vi "FTW-Collection-KeyValue-JSON-Serialize.vi"(1 "Key-Value Pair":T1) -> (0 "Serialized Key-Value Pair":string)   [LabVIEW 2014]
uses:
  FTW-Collection-KeyValuePair.ctl
  JSON/FTW-JSON-Escape.vi
panel:
  # "Inputs"
  # "Outputs"
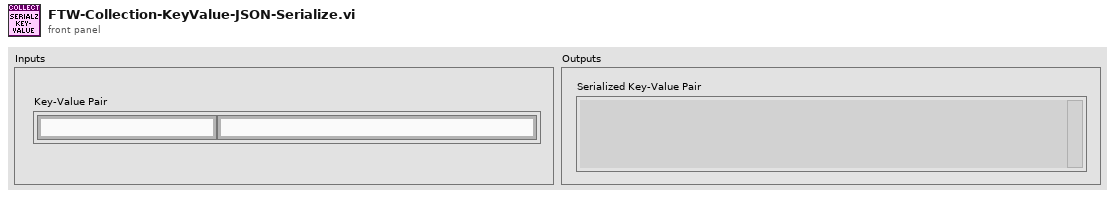
[diagram p1: front panel]
types:
  T1 = typedef "FTW-Collection-KeyValuePair.ctl" = cluster{"Key":string, "Value":string}
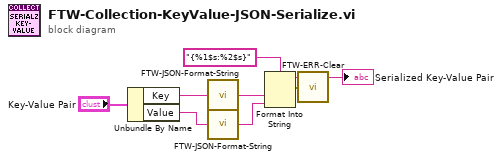
[diagram p0: block diagram]
diagram:
  n1 = Unbundle By Name("Key-Value Pair") -> ("Key"=w5:string, "Value"=w4:string)
  n2 = call "FTW-JSON-Format-String.vi"("LabVIEW String"=w5) -> ("JSON String"=w8:string)
  n3 = call "FTW-JSON-Format-String.vi"("LabVIEW String"=w4) -> ("JSON String"=w7:string)
  n4 = Format Into String(format string="{%1$s:%2$s}", w8, w7) -> (resulting string=→"Serialized Key-Value Pair":string, error out=w1:errorcluster)  [unwired: 2 in]
  n5 = call "FTW-ERR-Clear.vi"("error to snuff"=w1) -> ()  [unwired: 1 out]
